vi "HEWH Update Message.vi"(0 "Display Data (RLT) A":T1 {"Current Display" format="%.2f"; "Cycle Count Display" format="%04d"}, 1 "Test CompleteA":bool, 2 "Test CompleteB":bool, 3 "Test CompleteC":bool, 4 "Test CompleteD":bool, 5 "Display Data (RLT) B":T1 {"Current Display" format="%.2f"; "Cycle Count Display" format="%04d"}, 7 "Display Data (RLT) C":T1 {"Current Display" format="%.2f"; "Cycle Count Display" format="%04d"}, 9 "Display Data (RLT) D":T1 {"Current Display" format="%.2f"; "Cycle Count Display" format="%04d"}, 11 "error in (no error)":errorcluster) -> (15 "error out":errorcluster)   [LabVIEW 2019]
uses:
  Utility/Save File/Public/Type Definitions/Save File Appliance Display.ctl
  Utility/Save File/Public/Type Definitions/Save File Unit Type.ctl
  Utility/Save File/Save File.lvlib
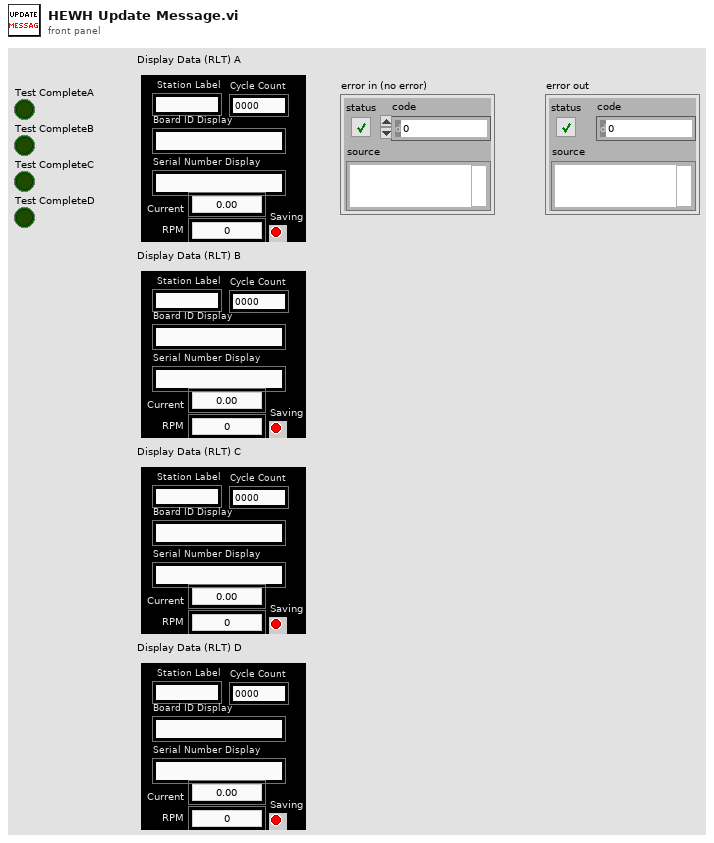
[diagram p1: front panel]
types:
  T1 = typedef "Save File Appliance Display.ctl" = cluster{"Status Color":u32, "Serial Number Display":string, "Cycle Count Display":i32, "Station Label Display":string, "Current Run Start Time Display":dbl, "Board ID Display":string, "RPM Display":u32, "Current Display":dbl, "Current Path Display":path, "Saving Display":bool, "Unit Type Display":T2, "Total Time On Display":dbl, "UI Button":bool}
  T2 = typedef "Save File.lvlib/Save File Unit Type.ctl" = enum32{"", "Viper", "Hawk", "2015"}
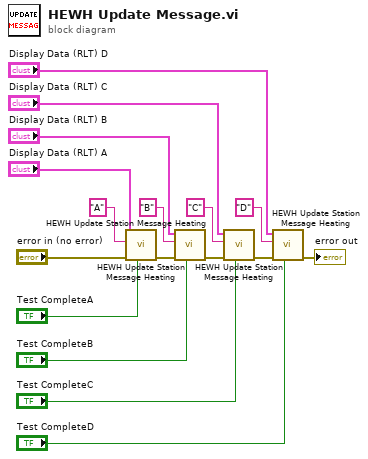
[diagram p0: block diagram]
diagram:
  n1 = call "HEWH Update Station Message Heating.vi"("Test Complete"="Test CompleteA", "error in (no error)"="error in (no error)", "Station Label"="A", "Display Data (RLT)"="Display Data (RLT) A") -> ("error out"=w12:errorcluster)  [unwired: 7 in]
  n2 = call "HEWH Update Station Message Heating.vi"("Test Complete"="Test CompleteB", "error in (no error)"=w12, "Station Label"="B", "Display Data (RLT)"="Display Data (RLT) B") -> ("error out"=w11:errorcluster)  [unwired: 7 in]
  n3 = call "HEWH Update Station Message Heating.vi"("Test Complete"="Test CompleteC", "error in (no error)"=w11, "Station Label"="C", "Display Data (RLT)"="Display Data (RLT) C") -> ("error out"=w10:errorcluster)  [unwired: 7 in]
  n4 = call "HEWH Update Station Message Heating.vi"("Test Complete"="Test CompleteD", "error in (no error)"=w10, "Station Label"="D", "Display Data (RLT)"="Display Data (RLT) D") -> ("error out"=→"error out":errorcluster)  [unwired: 7 in]
